vi "SubPanel - Frequency Domain Analysis.vi"() -> ()   [LabVIEW 2021]
uses:
  <vilib>/Analysis/4window.llb/windowTd.ctl
  <vilib>/measure/matone.llb/Harmonic Distortion Analyzer 1 Chan.vi
  <vilib>/measure/NI_MAPro.lvlib
  <vilib>/Analysis/NI_AALPro.lvlib
panel:
  out "error out":errorcluster
  in  "error in":errorcluster
  in  "Samples per Channel":i32
  out "Harmonic Levels":cluster{"Order":dbl, "RMS Level":dbl}[](array[cluster]) {"RMS Level" format="%#_6f"}
  out "Frequency Domain Signal (FFT Spectrum)":dbl[](graph) caption="Time Domain Signal"
  out "Time Domain Signal":waveform(dbl)[](graph)
  in  "Window":T1 items=["Rectangle", "Hanning", "Hamming", "Blackman-Harris", "Exact Blackman", "Blackman", "Flat Top", "4 Term B-Harris ", "7 Term B-Harris", "Low Sidelobe", "Blackman Nuttall", "Triangle", "Bartlett-Hanning", "Bohman", "Parzen", "Welch", "Kaiser", "Dolph-Chebyshev", "Gaussian"]
  in  "FFT Size":i32
  out "Detected Fundamental Frequency":dbl
  out "THD":dbl format="%#_6f"
  in  "Signal Selection":T2(radio)
  out "Harmonics":cluster{"X":dbl, "Y":dbl}[](graph)
  # "Detected Fundamental Frequency"
  # "THD"
  # "Hz"
  # "%"
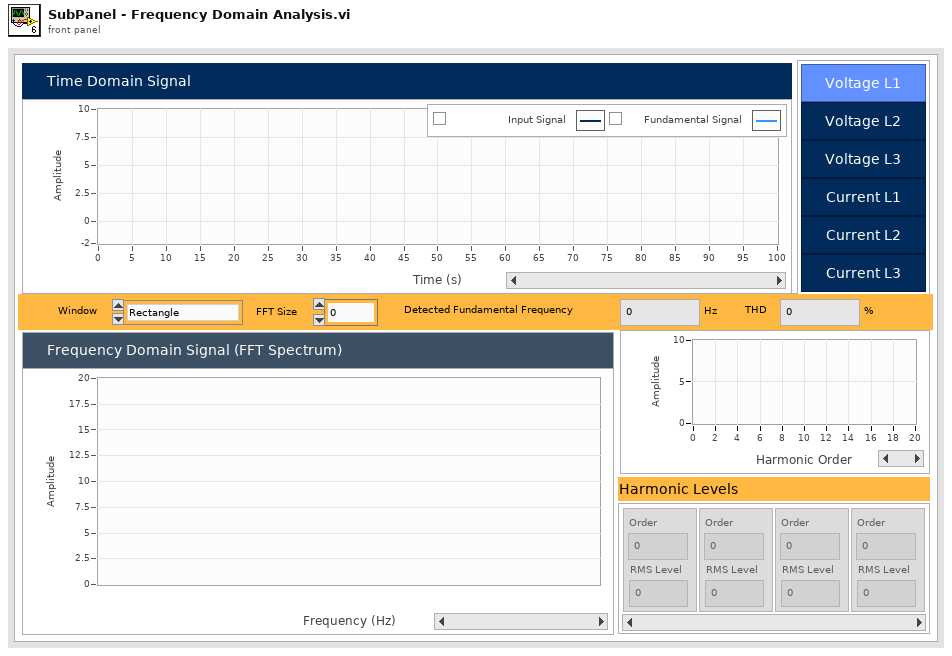
[diagram p1: front panel]
types:
  T1 = typedef "NI_AALPro.lvlib/windowTd.ctl" = u16
  T2 = enum32{"Button 1", "Button 2", "Button 3", "Button 4", "Button 5", "Button 6"}
  T3 = typedef "Message FPGA.ctl" = cluster{"Channel 1 Data (L1 U)":dbl[], "Channel 2 Data (L1 I)":dbl[], "Channel 3 Data (L2 U)":dbl[], "Channel 4 Data (L2 I)":dbl[], "Channel 5 Data (L3 U)":dbl[], "Channel 6 Data (L3 I)":dbl[]}
  T4 = enum16{"none", "input signal", "fundamental signal", "residual signal", "harmonics only", "noise and spurs"}
  T5 = cluster{"exported time signal":waveform(dbl), "exported spectrum (dB)":cluster{"f0":dbl, "df":dbl, "dB Spectrum (Hann)":dbl[]}}
  T6 = cluster{"f0":dbl, "df":dbl, "dB Spectrum (Hann)":dbl[]}
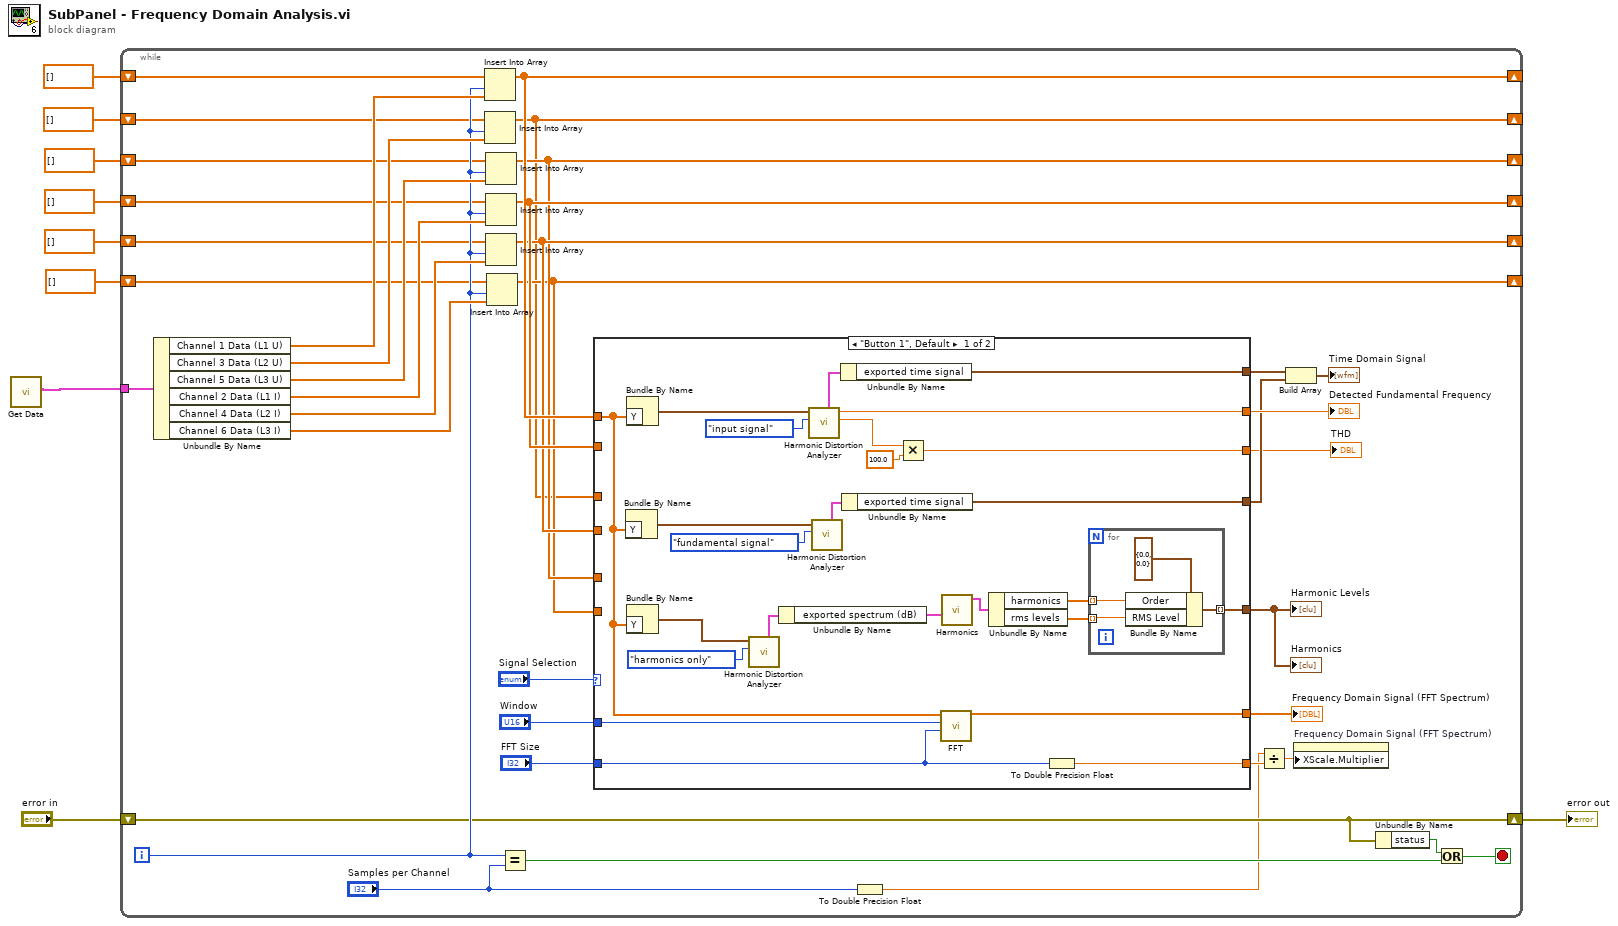
[diagram p0: block diagram]
diagram:
  n1 = call "Get Data.vi"() -> ("Message FPGA"=w1:T3)  [unwired: 10 in, 1 out]
  n2 = while {
    tunnel: w1 -> [w47]
    shift-right: [w28] -> _
    shift-left: dbl[] [] -> [w36]
    shift-right: [w11] -> _
    shift-left: dbl[] [] -> [w35]
    shift-right: [w25] -> _
    shift-left: dbl[] [] -> [w34]
    shift-right: [w27] -> _
    shift-left: dbl[] [] -> [w33]
    shift-right: [w26] -> _
    shift-left: dbl[] [] -> [w32]
    shift-right: [w24] -> _
    shift-left: dbl[] [] -> [w31]
    shift-right: [w30] -> w2
    shift-left: "error in" -> [w30]
    i -> [w40]
    stop <- w39 stop-if-true
    n3 = Unbundle By Name(w47) -> ("Channel 1 Data (L1 U)"=w46:dbl[], "Channel 3 Data (L2 U)"=w45:dbl[], "Channel 5 Data (L3 U)"=w44:dbl[], "Channel 2 Data (L1 I)"=w43:dbl[], "Channel 4 Data (L2 I)"=w42:dbl[], "Channel 6 Data (L3 I)"=w41:dbl[])
    n4 = Insert Into Array(array=w36, index=w40, new element=w46) -> (w28:dbl[])
    n5 = Insert Into Array(array=w35, index=w40, new element=w45) -> (w11:dbl[])
    n6 = Insert Into Array(array=w34, index=w40, new element=w44) -> (w25:dbl[])
    n7 = Insert Into Array(array=w33, index=w40, new element=w43) -> (w27:dbl[])
    n8 = Insert Into Array(array=w32, index=w40, new element=w42) -> (w26:dbl[])
    n9 = Insert Into Array(array=w31, index=w40, new element=w41) -> (w24:dbl[])
    n10 = Equal?(x=w40, y="Samples per Channel") -> (x = y?=w37:bool)
    n11 = case shown="\"Button 1\", Default" "Signal Selection" {
      tunnel: w28 -> [w56 _]
      tunnel: w27 -> [_ _]
      tunnel: w11 -> [_ _]
      tunnel: w26 -> [_ _]
      tunnel: w25 -> [_ _]
      tunnel: w24 -> [_ _]
      tunnel: [w64 _] -> w21
      tunnel: [w63 _] -> w23
      tunnel: [w62 _] -> w20
      tunnel: [w61 _] -> w19
      tunnel: "Window" -> [w60 _]
      tunnel: "FFT Size" -> [w58 _]
      tunnel: [w59 _] -> w16
      tunnel: [w57 _] -> w14
      tunnel: [w49 _] -> w10
      frame "Button 1", Default {
        n12 = Bundle By Name("Y"=w56) -> (w67:waveform(dbl))  [unwired: 1 in]
        n13 = Bundle By Name("Y"=w56) -> (w68:waveform(dbl))  [unwired: 1 in]
        n14 = Bundle By Name("Y"=w56) -> (w55:waveform(dbl))  [unwired: 1 in]
        n15 = call-poly <vilib>:"Harmonic Distortion Analyzer.vi"("export mode"=T4."harmonics only", "signal in"=w55) -> ("exported signals"=w54:T5)  [unwired: 4 in, 5 out]
        n16 = Unbundle By Name(w54) -> ("exported spectrum (dB)"=w48:T6)
        n17 = call-poly <vilib>:"Harmonic Distortion Analyzer.vi"("export mode"=T4."input signal", "signal in"=w68) -> ("THD"=w72:dbl, "detected fundamental frequency"=w63:dbl, "exported signals"=w69:T5)  [unwired: 4 in, 3 out]
        n18 = call-poly <vilib>:"Harmonic Distortion Analyzer.vi"("export mode"=T4."fundamental signal", "signal in"=w67) -> ("exported signals"=w66:T5)  [unwired: 4 in, 5 out]
        n19 = Unbundle By Name(w69) -> ("exported time signal"=w64:waveform(dbl))
        n20 = Unbundle By Name(w66) -> ("exported time signal"=w62:waveform(dbl))
        n21 = Multiply(x=w72, y=100.0) -> (x*y=w61:dbl)
        n22 = call "FFT.vi"("FFT size"=w58, "Window"=w60, "Time Domain Signal"=w56) -> ("Frequency Domain Signal"=w59:dbl[])  [unwired: 7 in, 1 out]
        n23 = call "Harmonics.vi"("complex spectrum"=w48) -> ("harmonic levels"=w50:cluster{"harmonics":dbl[], "rms levels":dbl[]})  [unwired: 8 in, 2 out]
        n24 = Unbundle By Name(w50) -> ("harmonics"=w52:dbl[], "rms levels"=w51:dbl[])
        n25 = To Double Precision Float(number=w58) -> (double precision float=w57:dbl)
        n26 = for {
          tunnel: w52 -> [w75] mode=indexing
          tunnel: w51 -> [w74] mode=indexing
          tunnel: [w73] -> w49 mode=indexing
          n27 = Bundle By Name(cluster=cluster{"Order":dbl, "RMS Level":dbl} {"Order"=0.0, "RMS Level"=0.0} ("Harmonics Levels"), "Order"=w75, "RMS Level"=w74) -> (w73:cluster{"Order":dbl, "RMS Level":dbl})
        }
      }
      frame "Button 2" {
      }
    }
    "Detected Fundamental Frequency" <- w23
    "THD" <- w19
    "Harmonics" <- w10
    "Harmonic Levels" <- w10
    "Frequency Domain Signal (FFT Spectrum)" <- w16
    n28 = To Double Precision Float(number="Samples per Channel") -> (double precision float=w12:dbl)
    n29 = Divide(x=w12, y=w14) -> (x/y=w15:dbl)
    n30 = Build Array(w21, w20) -> (→"Time Domain Signal":waveform(dbl)[])
    n31 = property on="Frequency Domain Signal (FFT Spectrum)" class="WFGraph (strict)"("XScale.Multiplier"=w15) -> ()  [unwired: 2 in, 2 out]
    n32 = Unbundle By Name(w30) -> ("status"=w38:bool)
    n33 = Or(x=w38, y=w37) -> (x .or. y?=w39:bool)
  }
  "error out" <- w2
